vi "Zaber A Series Frequency Control Cycling.vi"() -> ()   [LabVIEW 2012]
doc: "Shows a method of continuously cycling a single device based on timing (frequency). Demonstrates various library VIs such as Move, Set Speed and Accel, Home, and Request."
uses:
  <instrlib>/Zaber A Series/Zaber A Series.lvlib
panel:
  in  "Device and Axis":string
  in  "Distance Units (0: microsteps)":u16(ring) items=["microsteps", "microns", "millimeters", "inches"]
  in  "Speed/Accel Units (0: data)":u16(ring) items=["data", "microns/s, microns/s^2", "mm/s, mm/s^2", "inches/s, inches/s^2"]
  in  "New Speed (0)":dbl
  in  "New Accel (0)":dbl
  in  "Microstep Size (0)":dbl
  in  "VISA resource name":refnum<visa-resource-name>
  in  "Stop Cycling":bool
  in  "Frequency (Hz)":dbl=1.0
  in  "Starting Position":dbl
  # "(c) 2014 Zaber Technologies.  ALL RIGHTS RESERVED."
  # "There are a number of ways you can use Zaber devices to cycle or generate a frequency. This example shows one way that should have accurate cycle time. It used the 'move vel' command based on the input speed, and alternates directions through a Sequence Frame structure with wait commands to generate the correct timing. The downside of this method is that you need to use the Accel and Speed settings to adjust the amplitude of the cycles. Adjusting the accel value will also adjust the shape of the cycle."
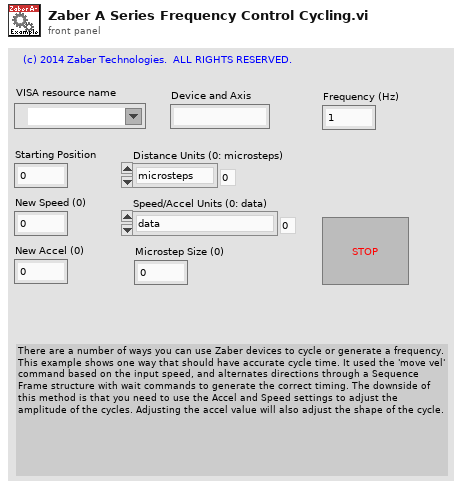
[diagram p1: front panel]
types:
  T1 = cluster{"Device":string, "Axis":string, "Reply Flag":string, "Status":string, "Warning Flags":string, "Data":string}[]
  T2 = cluster{"Device":string, "Axis":string, "Reply Flag":string, "Status":string, "Warning Flags":string, "Data":string}
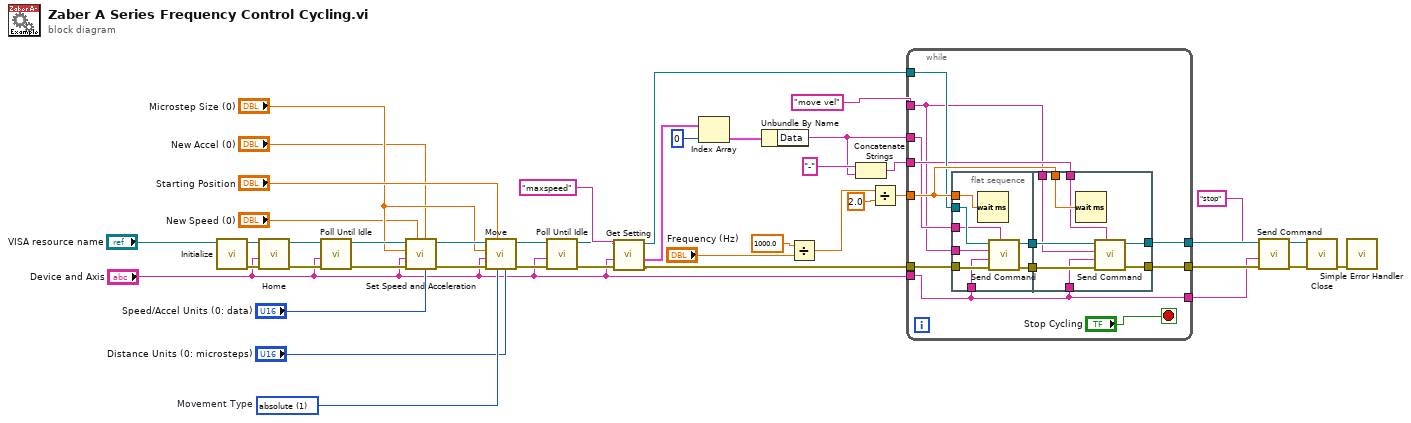
[diagram p0: block diagram]
diagram:
  w21 = u16 1 items=["relative", "absolute"]  # Movement Type
  n1 = call <instrlib>:"Initialize.vi"("VISA resource name"="VISA resource name") -> ("error out"=w24:errorcluster, "VISA resource name out"=w25:refnum<visa-resource-name>)  [unwired: 9 in]
  n2 = call <instrlib>:"Home.vi"("error in (no error)"=w24, "Device and Axis"="Device and Axis", "VISA resource name"=w25) -> ("error out"=w22:errorcluster, "VISA resource name out"=w28:refnum<visa-resource-name>)  [unwired: 7 in]
  n3 = call <instrlib>:"Poll Until Idle.vi"("error in (no error)"=w22, "Device and Axis"="Device and Axis", "VISA resource name"=w28) -> ("error out"=w26:errorcluster, "VISA resource name out"=w27:refnum<visa-resource-name>)  [unwired: 7 in]
  n4 = call <instrlib>:"Set Speed and Acceleration.vi"("Units (0: data)"="Speed/Accel Units (0: data)", "New Acceleration (0)"="New Accel (0)", "New Speed (0)"="New Speed (0)", "error in (no error)"=w26, "Device and Axis"="Device and Axis", "Microstep Size (0)"="Microstep Size (0)", "VISA resource name"=w27) -> ("error out"=w42:errorcluster, "VISA resource name out"=w43:refnum<visa-resource-name>)  [unwired: 3 in]
  n5 = call <instrlib>:"Move.vi"("Units (0: microsteps)"="Distance Units (0: microsteps)", "Movement Type (0: relative)"=w21, "Move Distance (0)"="Starting Position", "error in (no error)"=w42, "Device and Axis"="Device and Axis", "Microstep Size (0)"="Microstep Size (0)", "VISA resource name"=w43) -> ("error out"=w39:errorcluster, "VISA resource name out"=w40:refnum<visa-resource-name>)  [unwired: 3 in]
  n6 = call <instrlib>:"Poll Until Idle.vi"("error in (no error)"=w39, "Device and Axis"="Device and Axis", "VISA resource name"=w40) -> ("error out"=w18:errorcluster, "VISA resource name out"=w19:refnum<visa-resource-name>)  [unwired: 7 in]
  n7 = call <instrlib>:"Get Setting.vi"("error in (no error)"=w18, "Device and Axis"="Device and Axis", "Setting"="maxspeed" ("Common Settings"), "VISA resource name"=w19) -> ("error out"=w15:errorcluster, "Response Bundle Array"=w16:T1, "VISA resource name out"=w17:refnum<visa-resource-name>)  [unwired: 3 in, 2 out]
  n8 = Index Array(array=w16, index=0) -> (element=w37:T2)
  n9 = Unbundle By Name(w37) -> ("Data"=w14:string)
  n10 = Divide(x=1000.0, y="Frequency (Hz)") -> (x/y=w33:dbl)
  n11 = Concatenate Strings("-" ("string"), w14) -> (w30:string)
  n12 = Divide(x=w33, y=2.0) -> (x/y=w32:dbl)
  n13 = while {
    tunnel: [w54] -> w9
    tunnel: w32 -> [w53]
    tunnel: w17 -> [w52]
    tunnel: w15 -> [w51]
    tunnel: w30 -> [w49]
    tunnel: "Device and Axis" -> [w50]
    tunnel: [w50] -> w8
    tunnel: [w48] -> w10
    tunnel: w14 -> [w45]
    tunnel: "move vel" ("Complete Command List") -> [w44]
    stop <- "Stop Cycling" stop-if-true
    n14 = flat-sequence {
      tunnel: w53 -> [w63]
      tunnel: w52 -> [w62]
      tunnel: w51 -> [w59]
      tunnel: w44 -> [w56]
      tunnel: w50 -> [w58]
      tunnel: [w61] -> w47
      tunnel: [w60] -> w46
      tunnel: w45 -> [w57]
      tunnel: [w68] -> w54
      tunnel: w53 -> [w71]
      tunnel: w49 -> [w64]
      tunnel: w50 -> [w66]
      tunnel: [w69] -> w48
      tunnel: w47 -> [w70]
      tunnel: w46 -> [w67]
      tunnel: w44 -> [w65]
      frame #0 {
        n15 = Wait (ms)(milliseconds to wait=w63) -> ()  [unwired: 1 out]
        n16 = call <instrlib>:"Send Command.vi"("Data"=w57, "error in (no error)"=w59, "Device and Axis"=w58, "Command"=w56, "VISA resource name"=w62) -> ("error out"=w60:errorcluster, "VISA resource name out"=w61:refnum<visa-resource-name>)  [unwired: 2 in, 3 out]
      }
      frame #1 {
        n17 = Wait (ms)(milliseconds to wait=w71) -> ()  [unwired: 1 out]
        n18 = call <instrlib>:"Send Command.vi"("Data"=w64, "error in (no error)"=w67, "Device and Axis"=w66, "Command"=w65, "VISA resource name"=w70) -> ("error out"=w68:errorcluster, "VISA resource name out"=w69:refnum<visa-resource-name>)  [unwired: 2 in, 3 out]
      }
    }
  }
  n19 = call <instrlib>:"Send Command.vi"("error in (no error)"=w9, "Device and Axis"=w8, "Command"="stop" ("Complete Command List"), "VISA resource name"=w10) -> ("error out"=w11:errorcluster, "VISA resource name out"=w12:refnum<visa-resource-name>)  [unwired: 3 in, 3 out]
  n20 = call <instrlib>:"Close.vi"("error in (no error)"=w11, "VISA resource name"=w12) -> ("error out"=w23:errorcluster)  [unwired: 9 in]
  n21 = call <vilib>:"Simple Error Handler.vi"("error in (no error)"=w23) -> ()  [unwired: 4 in, 5 out]
